vi "FL_Decode_Serial_Stream_to_Coords.vi"(6 "Error In":errorcluster, 7 "Input timestamp":timestamp, 8 "Input string":string) -> (0 "Error Out":errorcluster, 1 "Full frame?":bool, 2 "Cluster of data":cluster{"alpha":dbl, "X":dbl, "Y":dbl}, 3 "Input string leftover":string)   [LabVIEW 2018]
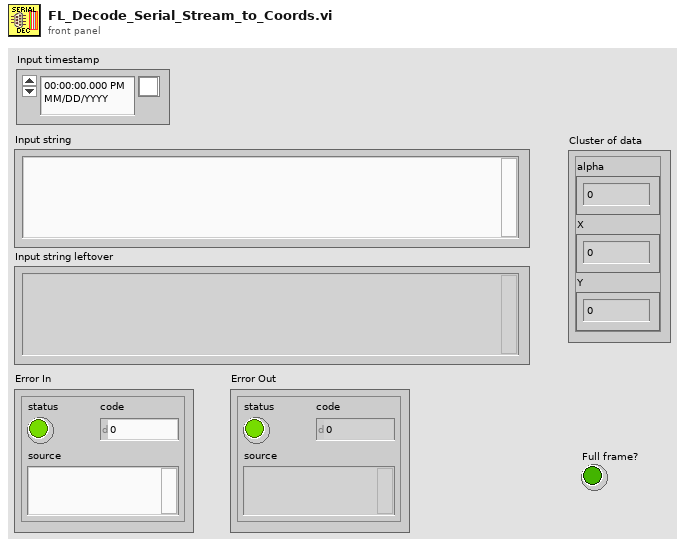
[diagram p1: front panel]
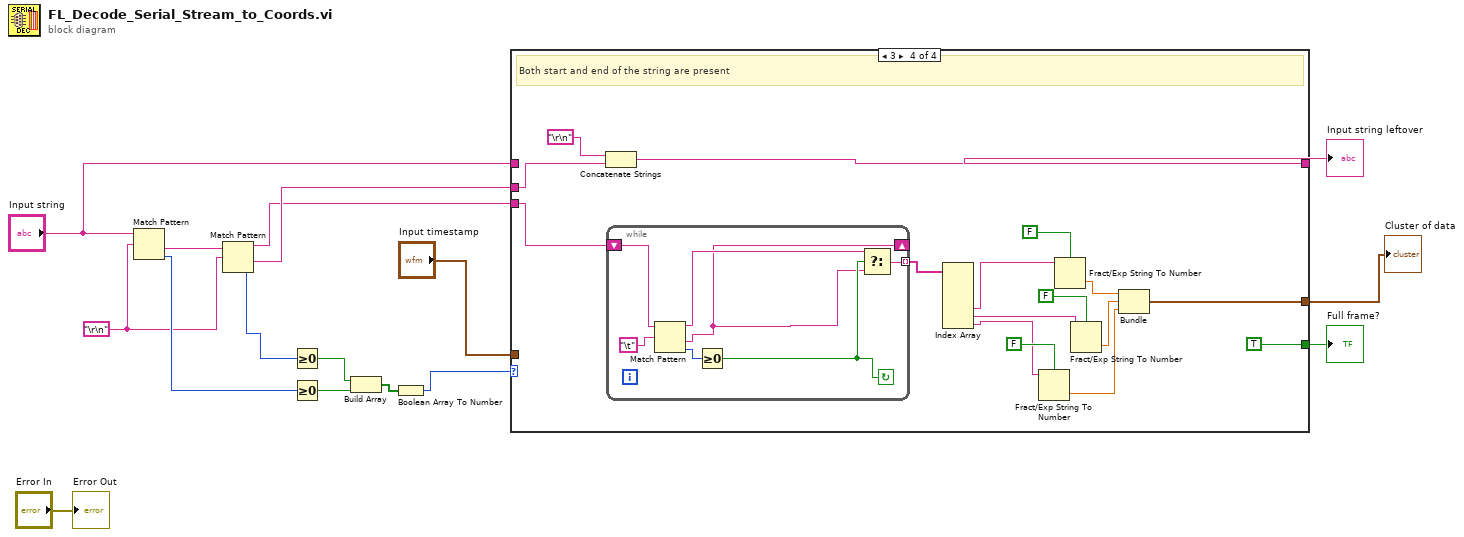
[diagram p0: block diagram]
diagram:
  w12 = "\r\n"
  n1 = Match Pattern(string="Input string", regular expression=w12) -> (after substring=w11:string, offset past match=w13:i32)  [unwired: 1 in, 2 out]
  n2 = Match Pattern(string=w11, regular expression=w12) -> (before substring=w3:string, after substring=w4:string, offset past match=w10:i32)  [unwired: 1 in, 1 out]
  n3 = Greater Or Equal To 0?(x=w10) -> (x >= 0?=w9:bool)
  n4 = Greater Or Equal To 0?(x=w13) -> (x >= 0?=w8:bool)
  n5 = Build Array(w9, w8) -> (w7:bool[])
  n6 = Boolean Array To Number(Boolean array=w7) -> (number=w6:u32)
  n7 = case shown="3" w6 {
    tunnel: "Input timestamp" -> [_ _ _ _]
    tunnel: "Input string" -> [w17 w18 w19 _]
    tunnel: [w17 w18 w19 w34] -> w5
    tunnel: w4 -> [_ _ _ w35]
    tunnel: w3 -> [_ _ _ w32]
    tunnel: [_ _ _ w21] -> w2
    tunnel: [_ _ _ TRUE] -> w1
    frame 0, Default {
      # "Nether start, not the end of the string is present"
    }
    frame 1 {
      # "Start of the string is present, but not the end"
    }
    frame 2 {
      # "End of the string is present, but not the start"
    }
    frame 3 {
      # "Both start and end of the string are present"
      n8 = Concatenate Strings("\r\n", w35) -> (w34:string)
      n9 = while {
        tunnel: [w39] -> w31 mode=indexing
        shift-right: [w36] -> _
        shift-left: w32 -> [w42]
        stop <- w37 continue-if-true
        n10 = Match Pattern(string=w42, regular expression="\t") -> (before substring=w38:string, after substring=w36:string, offset past match=w40:i32)  [unwired: 1 in, 1 out]
        n11 = Greater Or Equal To 0?(x=w40) -> (x >= 0?=w37:bool)
        n12 = Select(t=w38, s=w37, f=w36) -> (s? t:f=w39:string)
      }
      n13 = Index Array(array=w31) -> (element #4=w30:string, element #5=w25:string, element #6=w26:string)  [unwired: 6 in, 3 out]
      n14 = Fract/Exp String To Number(use system decimal point (T)=FALSE, string=w26) -> (number=w22:dbl)  [unwired: 2 in, 1 out]
      n15 = Fract/Exp String To Number(use system decimal point (T)=FALSE, string=w30) -> (number=w24:dbl)  [unwired: 2 in, 1 out]
      n16 = Fract/Exp String To Number(use system decimal point (T)=FALSE, string=w25) -> (number=w23:dbl)  [unwired: 2 in, 1 out]
      n17 = Bundle(w24, w23, w22) -> (w21:cluster{dbl, dbl, dbl})  [unwired: 1 in]
    }
  }
  "Input string leftover" <- w5
  "Cluster of data" <- w2
  "Full frame?" <- w1
  "Error Out" <- "Error In"
